vi "CFN61G_U8-to-B62-83_v1.vi"(11 "U8_Input":u8[](array[numeric])) -> (1 "Reserved":sgl[](array[numeric]), 2 "Tick_Counter":u16, 3 "Data Validity Time":u16[](array[numeric]))   [LabVIEW 2017]
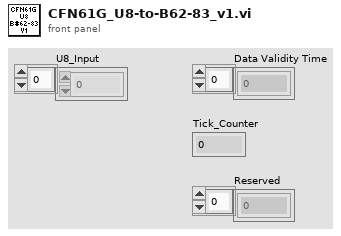
[diagram p1: front panel]
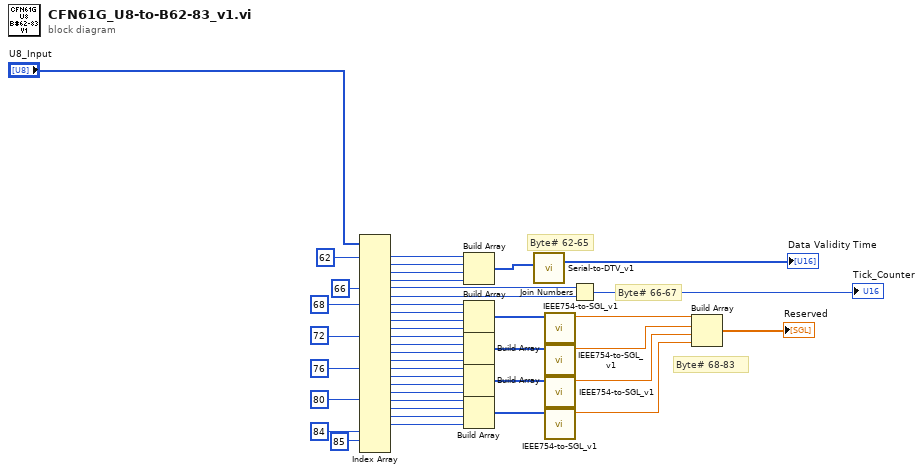
[diagram p0: block diagram]
diagram:
  # "Byte# 66-67"
  # "Byte# 62-65"
  # "Byte# 68-83"
  n1 = Index Array(array="U8_Input", index #1=62 ("index"), index #5=66 ("index"), index #7=68 ("index"), index #11=72 ("index"), index #15=76 ("index"), index #19=80 ("index"), index #23=84 ("index"), index #24=85 ("index")) -> (element #1=w39:u8, element #2=w40:u8, element #3=w41:u8, element #4=w42:u8, element #5=w36:u8, element #6=w37:u8, element #7=w13:u8, element #8=w14:u8, element #9=w15:u8, element #10=w16:u8, element #11=w17:u8, element #12=w18:u8, element #13=w19:u8, element #14=w20:u8, element #15=w21:u8, element #16=w22:u8, element #17=w23:u8, element #18=w24:u8, element #19=w25:u8, element #20=w26:u8, element #21=w27:u8, element #22=w28:u8)  [unwired: 17 in, 3 out]
  n2 = Build Array(w39, w40, w41, w42) -> (w10:u8[])
  n3 = Build Array(w13, w14, w15, w16) -> (w4:u8[])
  n4 = Build Array(w17, w18, w19, w20) -> (w1:u8[])
  n5 = Build Array(w21, w22, w23, w24) -> (w2:u8[])
  n6 = Build Array(w25, w26, w27, w28) -> (w3:u8[])
  n7 = call "Serial-to-DTV_v1.vi"("Input_U8"=w10) -> ("Data Validity Time"=→"Data Validity Time":u16[])  [unwired: 9 in, 1 out]
  n8 = call "IEEE754-to-SGL_v1.vi"("Input_U8"=w4) -> ("Output_SGL"=w6:sgl)  [unwired: 10 in]
  n9 = call "IEEE754-to-SGL_v1.vi"("Input_U8"=w1) -> ("Output_SGL"=w7:sgl)  [unwired: 10 in]
  n10 = call "IEEE754-to-SGL_v1.vi"("Input_U8"=w2) -> ("Output_SGL"=w8:sgl)  [unwired: 10 in]
  n11 = call "IEEE754-to-SGL_v1.vi"("Input_U8"=w3) -> ("Output_SGL"=w9:sgl)  [unwired: 10 in]
  n12 = Join Numbers(hi=w36, lo=w37) -> ((hi.lo)=→"Tick_Counter":u16)
  n13 = Build Array(w6, w7, w8, w9) -> (→"Reserved":sgl[])
